vi "Manage Background Music.vi"(8 "error in (no error)":errorcluster, 9 "Music Paused":bool, 10 "Application In":refnum<class "Application.lvclass">, 11 "Sounds":cluster{"Sound Effect":T1, "Task ID":T2}[](array[cluster]) {"Task ID" format="%.0x"}) -> (0 "error out":errorcluster, 3 "Sounds Out":cluster{"Sound Effect":T1, "Task ID":T2}[](array[cluster]) {"Task ID" format="%.0x"})   [LabVIEW 2021, in "Application.lvclass"]
uses:
  Application.lvclass
  Sound Effects.ctl
  <vilib>/sound2/lvsound2.llb/Sound Output Task ID.ctl
  Application.lvclass/Application.ctl
  <vilib>/numeric/Random Number (Range) DBL.vi
  <vilib>/sound2/lvsound2.llb/Sound Output Set Volume (Single).vi
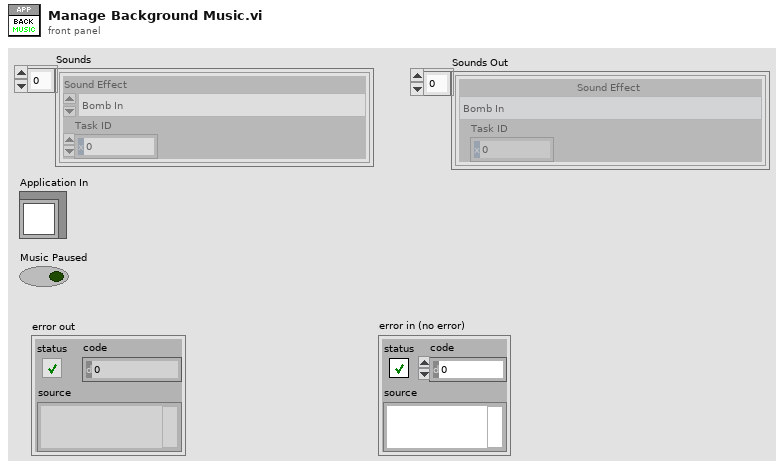
[diagram p1: front panel]
types:
  T1 = typedef "Application.lvclass/Sound Effects.ctl" = enum16{"Bomb In", "Bomb Out", "Bomb Touched", "Game Over", "Victory", "Eat", "10 Fruits", "Eat2", "Eat3", "Eat4", "MaxShield", "Shield", "10p", "Grape In", "Grape Out", "20p", "30p", "40p", "50p", "60p", "70p", "80p", "90p", "100p", "All shields cracked", "Mouse In", "Mouse Out", "Mouse Eaten", "Grape Eaten", "States Recover", "Broken Shield", "Bonus", "Happy Time", "explode", "Game over musica", "Back Music", "Shield Catch", "Evil lough", "Cricket In", "Cricket eaten", "Lets Go", "Jump1", "Jump2", "Jump3", "Unstoppable", "Troll Music", "winner"}
  T2 = typedef "Sound Output Task ID.ctl" = u32
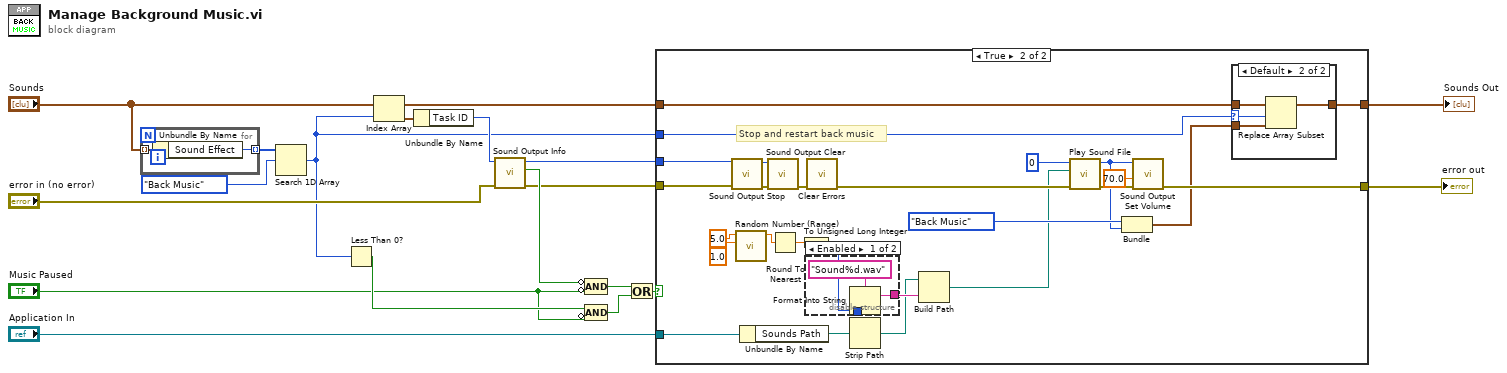
[diagram p0: block diagram]
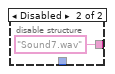
[diagram p3: hidden frame]
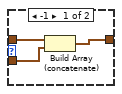
[diagram p4: hidden frame]
diagram:
  n1 = for {
    tunnel: "Sounds" -> [w20] mode=indexing
    tunnel: [w19] -> w15 mode=indexing
    n2 = Unbundle By Name(w20) -> ("Sound Effect"=w19:T1)
  }
  n3 = Search 1D Array(1D array=w15, element=Sound_Effects."Back Music") -> (index of element=w5:i32)  [unwired: 1 in]
  n4 = Less Than 0?(x=w5) -> (x < 0?=w4:bool)
  n5 = Index Array(array="Sounds", index=w5) -> (element=w17:cluster{"Sound Effect":T1, "Task ID":T2})
  n6 = Unbundle By Name(w17) -> ("Task ID"=w18:T2)
  n7 = call <vilib>:"Sound Output Info.vi"("error in (no error)"="error in (no error)", "task ID"=w18) -> ("error out"=w10:errorcluster, "is playing?"=w13:bool, "task ID out"=w11:T2)  [unwired: 6 in, 1 out]
  n8 = Compound Arithmetic op=AND(invert w13, invert "Music Paused") -> (w12:bool)
  n9 = Compound Arithmetic op=AND(w4, invert "Music Paused") -> (w1:bool)
  n10 = Or(x=w12, y=w1) -> (x .or. y?=w2:bool)
  n11 = case shown="True" w2 {
    tunnel: w11 -> [_ w46]
    tunnel: w10 -> [w21 w45]
    tunnel: "Sounds" -> [w22 w43]
    tunnel: "Application In" -> [_ w28]
    tunnel: [w21 w37] -> w6
    tunnel: w5 -> [_ w35]
    tunnel: [w22 w34] -> w7
    frame False {
    }
    frame True {
      # "Stop and restart back music"
      n12 = call <vilib>:"Sound Output Stop.vi"("error in (no error)"=w45, "task ID"=w46) -> ("error out"=w44:errorcluster, "task ID out"=w47:T2)  [unwired: 8 in]
      n13 = call-poly <vilib>:"Random Number (Range).vi"("lower bound (0)"=1.0 ("Low"), "upper bound (100)"=5.0 ("High")) -> ("number"=w31:dbl)  [unwired: 9 in]
      n14 = Unbundle By Name(w28) -> ("Sounds Path"=w26:path)
      n15 = call <vilib>:"Sound Output Clear.vi"("error in (no error)"=w44, "task ID"=w47) -> ("error out"=w48:errorcluster)  [unwired: 9 in]
      n16 = Round To Nearest(number=w31) -> (nearest integer value=w30:dbl)
      n17 = To Unsigned Long Integer(number=w30) -> (unsigned 32bit integer=w27:u32)
      n18 = disable-structure shown="Enabled" {
        disable-tunnel: w27 -> [w51 _]
        disable-tunnel: [w49 "Sound7.wav"] -> w25
        frame Enabled {
          n19 = Format Into String(format string="Sound%d.wav", w51) -> (resulting string=w49:string)  [unwired: 2 in, 1 out]
        }
        frame Disabled {
        }
      }
      n20 = call <vilib>:"Clear Errors.vi"("error in (no error)"=w48) -> ("error out"=w40:errorcluster)  [unwired: 5 in, 1 out]
      n21 = Strip Path(path=w26) -> (stripped path=w23:path)  [unwired: 1 out]
      n22 = Build Path(base path=w23, name or relative path=w25) -> (appended path=w24:path)
      n23 = call <vilib>:"Play Sound File.vi"("error in (no error)"=w40, "path"=w24, "device ID"=u32 0) -> ("error out"=w41:errorcluster, "task ID"=w38:T2)  [unwired: 7 in]
      n24 = Bundle("element"=Sound_Effects."Back Music", "task ID"=w38) -> (w36:cluster{"element":T1, "task ID":T2})  [unwired: 1 in]
      n25 = call-poly <vilib>:"Sound Output Set Volume.vi"("error in (no error)"=w41, "volume"=70.0, "task ID"=w38) -> ("error out"=w37:errorcluster)  [unwired: 7 in, 1 out]
      n26 = case shown="Default" w35 {
        selector: w35 -> [_ w57]
        tunnel: w43 -> [w55 w59]
        tunnel: w36 -> [w53 w58]
        tunnel: [w54 w56] -> w34
        frame -1 {
          n27 = Build Array (concatenate)(w55, w53) -> (w54:cluster{"element":T1, "task ID":T2}[])
        }
        frame Default {
          n28 = Replace Array Subset(array=w59, new element=w58, index=w57) -> (w56:cluster{"Sound Effect":T1, "Task ID":T2}[])
        }
      }
    }
  }
  "Sounds Out" <- w7
  "error out" <- w6
